vi "Run_Update_Functions2.vi"(3 "Debug Mode":bool, 4 "Time Delta (s)":dbl, 5 "API Function Array":cluster{string, "VI Reference":refnum<vi>}[](array[cluster]), 6 "Update Functions In":cluster{string, string[], dbl[], dbl}[](array[cluster])) -> (0 "Refresh":bool, 1 "Status Array":T1(array[cluster]), 2 "Update Functions Out":cluster{string, string[], dbl[], dbl}[](array[cluster]))   [LabVIEW 2011]
doc: "This VI will execute the appropriate dynamic API VI of all currently running functions during the main loop of a growth run. \"Time Delta (s)\" represents the amount of time in seconds since the last call to this VI. \"Status Array\" will output an array of function statuses from the updated functions, along with the appropriate argument lists to allow other SubVI's to determine the source of each status. \"Debug Mode\" disables all external hardware communications."
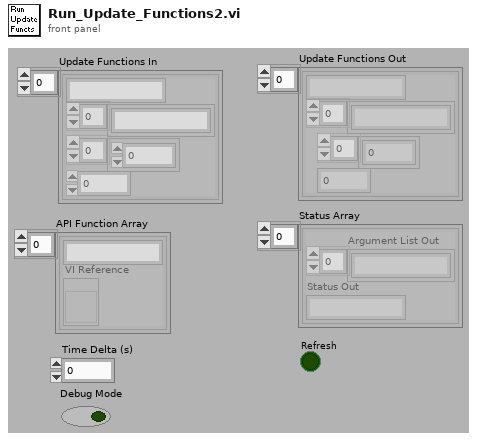
[diagram p1: front panel]
types:
  T1 = cluster{"Argument List Out":string[], "Status Out":string}[]
  T2 = cluster{string, "Argument List Out":string[], dbl[], dbl}
  T3 = enum16{"Discrete", "Continuous", "Instantaneous", "Finite"}
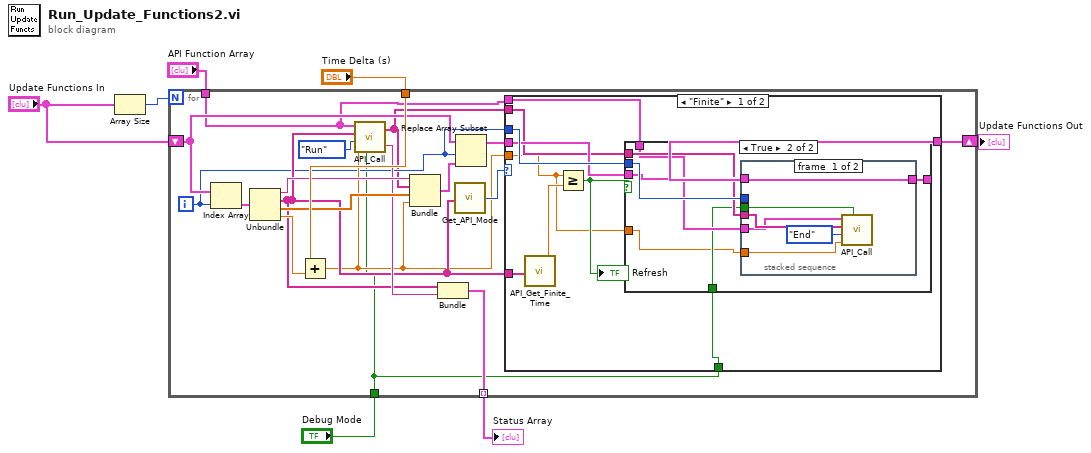
[diagram p0: block diagram]
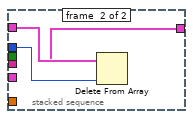
[diagram p3: hidden frame]
diagram:
  n1 = Array Size(array="Update Functions In") -> (size(s)=w7:i32)
  n2 = for {
    N: w7 -> [_]
    tunnel: "Time Delta (s)" -> [w25]
    tunnel: "Debug Mode" -> [w8]
    tunnel: [w17] -> w4 mode=indexing
    tunnel: "API Function Array" -> [w9]
    shift-right: [w16] -> w1
    shift-left: "Update Functions In" -> [w22]
    i -> [w11]
    n3 = Index Array(array=w22, index=w11) -> (element=w26:cluster{string, string[], dbl[], dbl})
    n4 = Unbundle(w26) -> (w24:string, w13:string[], w19:dbl[], w20:dbl)
    n5 = Add(x=w25, y=w20) -> (x+y=w12:dbl)
    n6 = call "API_Call.vi"("API Function Array"=w9, "Argument List In"=w13, "State"=enum16{"Edit", "Start", "Run", "End", "Idle"}."Run", "Elapsed Time (s)"=w12, "Debug Mode"=w8) -> ("Argument List Out"=w10:string[], "Status Out"=w18:string)
    n7 = Bundle(w24, "Argument List Out"=w10, w19, w12) -> (w23:T2)  [unwired: 1 out]
    n8 = Bundle(w13, "Status Out"=w18) -> (w17:cluster{string[], "Status Out":string})  [unwired: 1 out]
    n9 = call "Get_API_Mode.vi"("Argument List"=w13) -> ("API Mode"=w14:T3)
    n10 = Replace Array Subset(array=w22, new element=w23, index=w11) -> (w15:cluster{string, string[], dbl[], dbl}[])
    n11 = case shown="\"Finite\"" w14 {
      tunnel: [w34 w53] -> w16
      tunnel: w15 -> [w35 w53]
      tunnel: w13 -> [w33 _]
      tunnel: w12 -> [w27 _]
      tunnel: w11 -> [w36 _]
      tunnel: w10 -> [w30 _]
      tunnel: w9 -> [w29 _]
      tunnel: w8 -> [w28 _]
      frame "Finite" {
        n12 = call "API_Get_Finite_Time.vi"("Argument List"=w33) -> ("Finite Time"=w32:dbl)
        n13 = Greater Or Equal?(x=w27, y=w32) -> (x >= y?=w31:bool)
        "Refresh" <- w31
        n14 = case shown="True" w31 {
          tunnel: w36 -> [_ w44]
          tunnel: w35 -> [w37 w43]
          tunnel: [w37 w42] -> w34
          tunnel: w30 -> [_ w41]
          tunnel: w29 -> [_ w40]
          tunnel: w28 -> [_ w39]
          tunnel: w27 -> [_ w38]
          frame False {
          }
          frame True {
            n15 = stacked-sequence {
              tunnel: w44 -> [_ w52]
              tunnel: w43 -> [_ w51]
              tunnel: [_ w50] -> w42
              tunnel: w41 -> [w49 _]
              tunnel: w40 -> [w48 _]
              tunnel: w39 -> [w47 _]
              tunnel: w38 -> [w45 _]
              frame #0 {
                n16 = call "API_Call.vi"("API Function Array"=w48, "Argument List In"=w49, "State"=enum16{"Edit", "Start", "Run", "End", "Idle"}."End", "Elapsed Time (s)"=w45, "Debug Mode"=w47) -> ()  [unwired: 2 out]
              }
              frame #1 {
                n17 = Delete From Array(array=w51, index=w52) -> (array with subset deleted=w50:cluster{string, string[], dbl[], dbl}[])  [unwired: 1 in, 1 out]
              }
            }
          }
        }
      }
      frame Default {
      }
    }
  }
  "Update Functions Out" <- w1
  "Status Array" <- w4
